vi "main.vi"() -> ()   [LabVIEW 2024]
uses:
  Controls/#typedef_program_states_beer.ctl
  Controls/#typedef_program_data_beer.ctl
panel:
  out "error out":errorcluster
  in  "error in (no error)":errorcluster
  in  "Draught level [ml]":dbl(slide)=1.0 min=1.0 max=50.0 step=1.0 scale=1.0..50.0
  in  "No more drinking":bool
  in  "Drink beer":bool
  out "Beer slide":dbl(slide) scale=0.0..500.0
  in  "Cluster":T1 {"Draught level [ml]" scale=1.0..50.0; "Beer slide" scale=0.0..100.0}
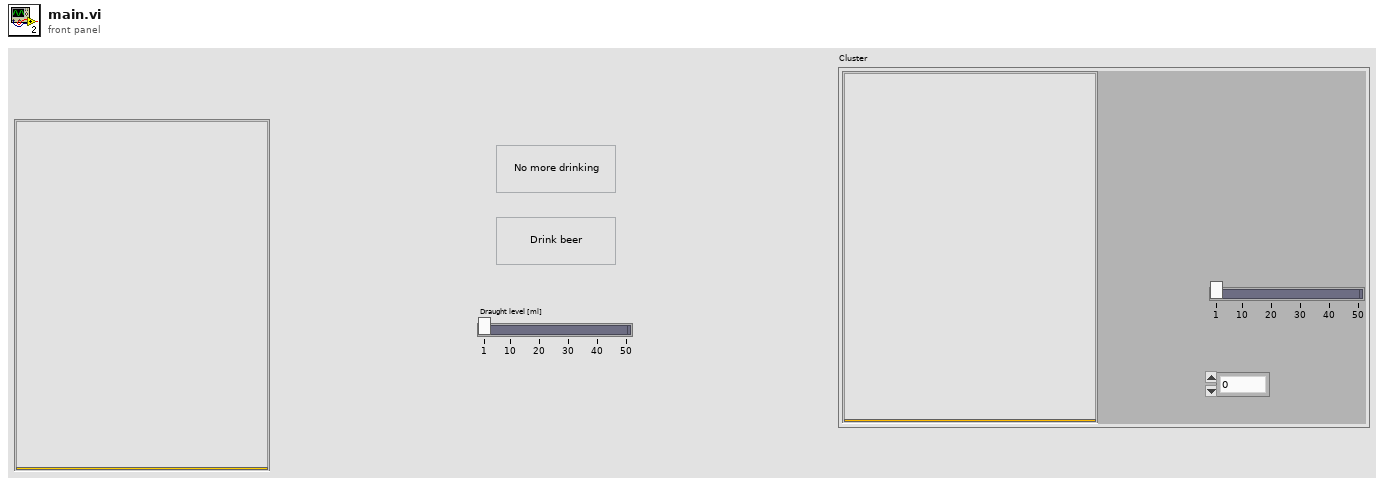
[diagram p1: front panel]
types:
  T1 = typedef "#typedef_program_data_beer.ctl" = cluster{"Beer slide":dbl, "Draught level [ml]":dbl, "beer number":dbl}
  T2 = typedef "#typedef_program_states_beer.ctl" = enum16{"application error", "init", "idle", "drink beer", "stop"}
  T3 = enum8{"Enabled", "Disabled", "Disabled and Grayed Out"}
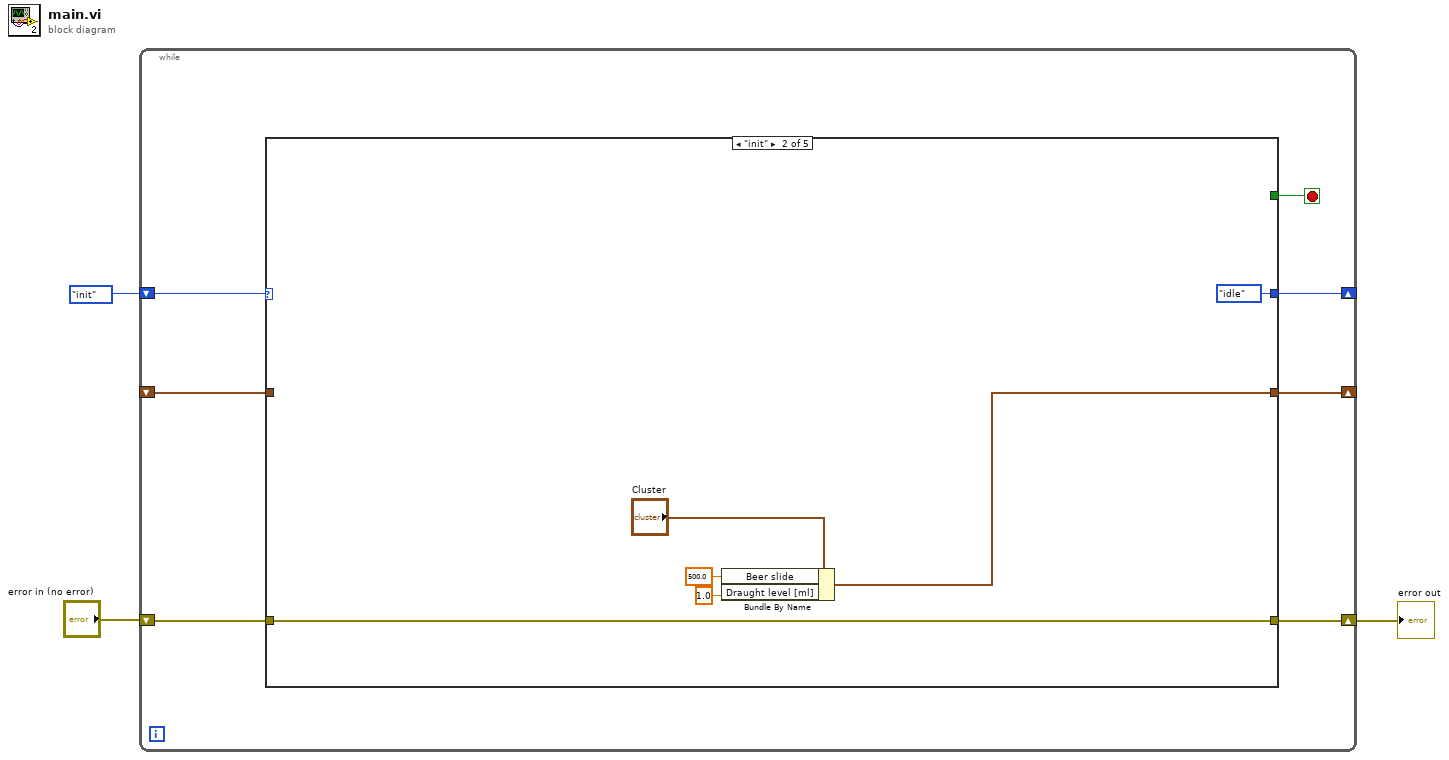
[diagram p0: block diagram]
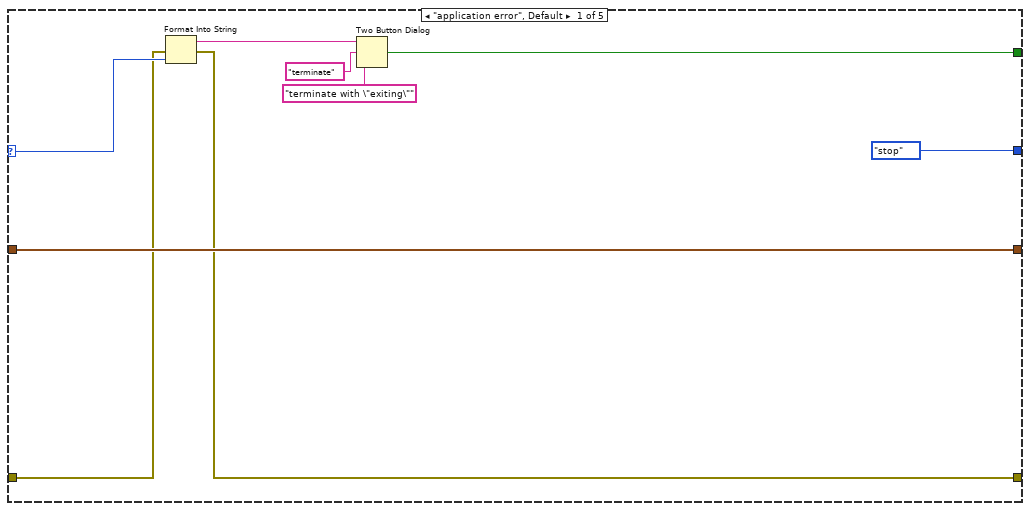
[diagram p2: hidden frame]
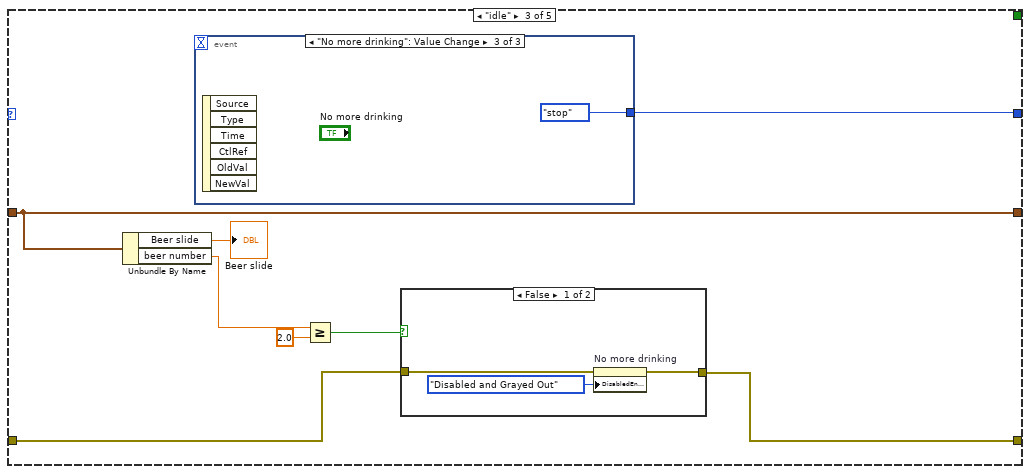
[diagram p3: hidden frame]
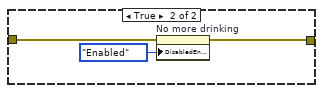
[diagram p4: hidden frame]
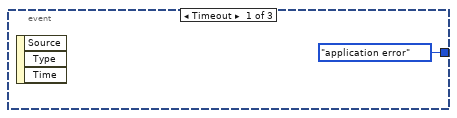
[diagram p5: hidden frame]
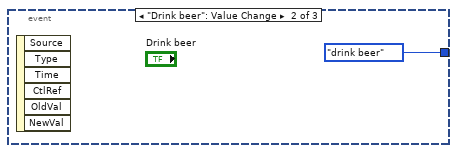
[diagram p6: hidden frame]
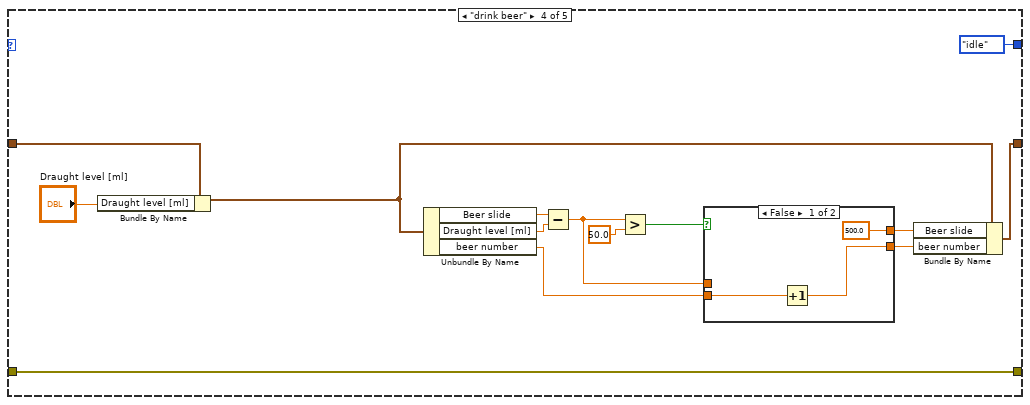
[diagram p7: hidden frame]
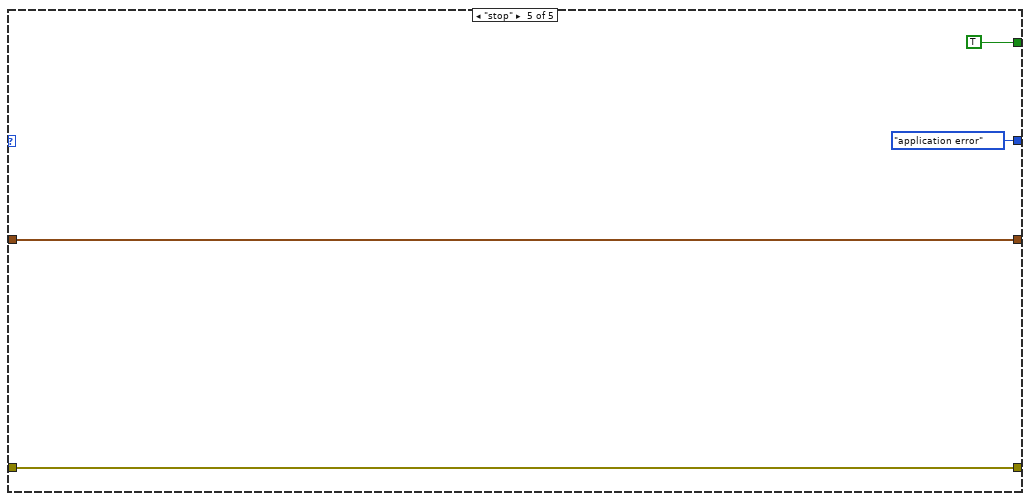
[diagram p9: hidden frame]
diagram:
  n1 = while {
    shift-right: [w8] -> _
    shift-left: #typedef_program_states_beer."init" ("program states beer") -> [w10]
    shift-right: [w7] -> _
    shift-left: _ -> [w6]
    shift-right: [w4] -> w1
    shift-left: "error in (no error)" -> [w5]
    stop <- w9 stop-if-true
    n2 = case shown="\"init\"" w10 {
      selector: w10 -> [w19 _ _ _ _]
      tunnel: [w15 _ _ _ TRUE] -> w9
      tunnel: [#typedef_program_states_beer."stop" ("program states beer") #typedef_program_states_beer."idle" ("program states beer") w33 #typedef_program_states_beer."idle" ("program states beer") #typedef_program_states_beer."application error" ("program states beer")] -> w8
      tunnel: [w13 w23 w31 w53 w63] -> w7
      tunnel: w6 -> [w13 _ w31 w52 w63]
      tunnel: w5 -> [w12 w20 w27 w43 w62]
      tunnel: [w11 w20 w26 w43 w62] -> w4
      frame "application error", Default {
        n3 = Format Into String(error in=w12, w19) -> (resulting string=w18:string, error out=w11:errorcluster)  [unwired: 2 in]
        n4 = Two Button Dialog(message=w18, 1:"terminate with \"exiting\"" ("F button name (\"Cancel\")"), 2:"terminate" ("T button name (\"OK\")")) -> (T button?=w15:bool)
      }
      frame "init" {
        n5 = Bundle By Name(cluster="Cluster", "Beer slide"=500.0, "Draught level [ml]"=1.0) -> (w23:T1)
      }
      frame "idle" {
        n6 = Unbundle By Name(w31) -> ("Beer slide"=→"Beer slide":dbl, "beer number"=w29:dbl)
        n7 = event shown="[2] \"No more drinking\": Value Change" {
          selector: _ -> [_ _ _]
          dyn-events: _ -> [_ _ _]
          timeout: _ -> [_ _ _]
          tunnel: [#typedef_program_states_beer."application error" ("program states beer") #typedef_program_states_beer."drink beer" ("program states beer") #typedef_program_states_beer."stop" ("program states beer")] -> w33
          event Timeout {
            n8 = event-data() -> ()  [unwired: 1 in, 3 out]
          }
          event "Drink beer": Value Change {
            n9 = event-data() -> ()  [unwired: 1 in, 6 out]
          }
          event "No more drinking": Value Change {
            n10 = event-data() -> ()  [unwired: 1 in, 6 out]
          }
        }
        n11 = Greater Or Equal?(x=w29, y=2.0) -> (x >= y?=w30:bool)
        n12 = case shown="False" w30 {
          tunnel: w27 -> [w35 w37]
          tunnel: [w34 w38] -> w26
          frame False {
            n13 = property on="No more drinking" class="Bool"(error in=w35, "DisabledEnum"=T3."Disabled and Grayed Out" ("Disabled")) -> (error out=w34:errorcluster)  [unwired: 1 in, 1 out]
          }
          frame True {
            n14 = property on="No more drinking" class="Bool"(error in=w37, "DisabledEnum"=T3."Enabled" ("Disabled")) -> (error out=w38:errorcluster)  [unwired: 1 in, 1 out]
          }
        }
      }
      frame "drink beer" {
        n15 = Bundle By Name(cluster=w52, "Draught level [ml]"="Draught level [ml]") -> (w51:T1)
        n16 = Unbundle By Name(w51) -> ("Beer slide"=w55:dbl, "Draught level [ml]"=w54:dbl, "beer number"=w45:dbl)
        n17 = Subtract(x=w55, y=w54) -> (x-y=w47:dbl)
        n18 = Greater?(x=w47, y=50.0) -> (0:w48:bool)
        n19 = case shown="False" w48 {
          tunnel: w47 -> [_ w61]
          tunnel: [500.0 ("f") w61] -> w46
          tunnel: w45 -> [w58 w60]
          tunnel: [w57 w60] -> w44
          frame False {
            n20 = Increment(x=w58) -> (x+1=w57:dbl)
          }
          frame True {
          }
        }
        n21 = Bundle By Name(cluster=w51, "Beer slide"=w46, "beer number"=w44) -> (w53:T1)
      }
      frame "stop" {
      }
    }
  }
  "error out" <- w1
